vi "Calibración Motores.vi"() -> ()   [LabVIEW 2016]
uses:
  <vilib>/LabVIEW Interface for Arduino/Type Defs/Board Type.ctl
  <vilib>/LabVIEW Interface for Arduino/LabVIEW Interface for Arduino.lvlib
panel:
  in  "X":dbl(slide) scale=0.0..90.0
  in  "Y":dbl(slide) scale=0.0..90.0
  in  "stop":bool
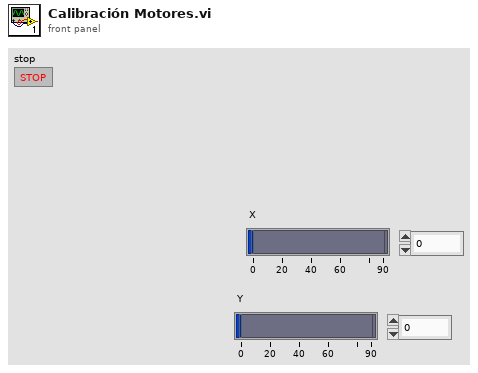
[diagram p1: front panel]
types:
  T1 = typedef "LabVIEW Interface for Arduino.lvlib/Board Type.ctl" = enum16{"Uno", "Dimuelanove w/Atmega 328", "Mega 2560"}
  T2 = typedef "LabVIEW Interface for Arduino.lvlib/Arduino Resource.ctl" = cluster{"VISA resource":refnum<visa-resource-name>, "Board Type":T1, "Connection Type":enum8{"USB / Serial"}, "Bytes Per Packet (15)":u8}
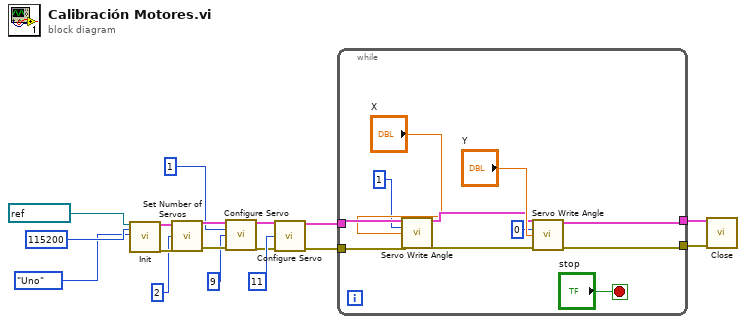
[diagram p0: block diagram]
diagram:
  n1 = call <vilib>:"Init.vi"("VISA resource"=refnum<visa-resource-name> "COM3", "Baud Rate (115200)"=u32 115200, "Board Type (Uno)"=Board_Type."Uno") -> ("Arduino Resource"=w17:T2, "error out"=w16:errorcluster)  [unwired: 15 in]
  n2 = call <vilib>:"Set Number of Servos.vi"("Arduino Resource"=w17, "Number Of Servos (1)"=u8 2, "error in"=w16) -> ("Arduino Resource"=w8:T2, "error out"=w7:errorcluster)  [unwired: 11 in]
  n3 = call <vilib>:"Configure Servo.vi"("Arduino Resource"=w8, "Servo Number (0)"=u8 1, "DIO Pin (2)"=u8 9, "error in"=w7) -> ("Arduino Resource"=w10:T2, "error out"=w9:errorcluster)  [unwired: 10 in]
  n4 = call <vilib>:"Configure Servo.vi"("Arduino Resource"=w10, "DIO Pin (2)"=u8 11, "error in"=w9) -> ("Arduino Resource"=w14:T2, "error out"=w13:errorcluster)  [unwired: 11 in]
  n5 = while {
    tunnel: w14 -> [w22]
    tunnel: w13 -> [w23]
    tunnel: [w26] -> w12
    tunnel: [w27] -> w11
    stop <- "stop" stop-if-true
    n6 = call <vilib>:"Servo Write Angle.vi"("Arduino Resource"=w22, "Servo Number"=u8 1, "Angle (Degrees)"="X", "error in"=w23) -> ("Arduino Resource"=w21:T2, "error out"=w20:errorcluster)  [unwired: 10 in]
    n7 = call <vilib>:"Servo Write Angle.vi"("Arduino Resource"=w21, "Servo Number"=u8 0, "Angle (Degrees)"="Y", "error in"=w20) -> ("Arduino Resource"=w26:T2, "error out"=w27:errorcluster)  [unwired: 10 in]
  }
  n8 = call <vilib>:"Close.vi"("Arduino Resource"=w12, "error in"=w11) -> ()  [unwired: 13 in, 1 out]
